vi "subvi.vi"(11 "F":dbl) -> (3 "Numeric":dbl)   [LabVIEW 2018]
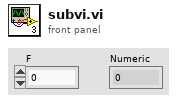
[diagram p1: front panel]
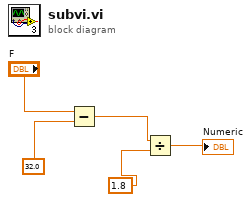
[diagram p0: block diagram]
diagram:
  n1 = Subtract(x="F", y=32.0) -> (x-y=w3:dbl)
  n2 = Divide(x=w3, y=1.8) -> (x/y=→"Numeric":dbl)
